vi "CAN Alerts.vi"(10 "RobotDriveDevRef":T1={"DevStatus"={"status"=FALSE, "code"=0, "source"=""}, "Motors[]"=[], "Square Inputs"=FALSE, "Max Output"=1.0}, 11 "CAN Talon List":string[](array[string])) -> ()   [LabVIEW 2014, in "hhVI.lvlib"]
doc: "Checks voltage of the PDV, roboRIO and all CAN Talon motor controllers. If the voltage on any of these it too low a dashboard message \"Voltage Alerts\" is sent."
uses:
  hhVI.lvlib
  <vilib>/Rock Robotics/Network Tables/SD Write String.vi
  <vilib>/Rock Robotics/WPI/PWM/WPI_PWMTransform_ConPane.ctl
  <vilib>/Rock Robotics/WPI/CAN/Jaguar/SubVIs/WPI_CANJaguar_ControlMode.ctl
  <vilib>/Rock Robotics/WPI/CAN/TalonSRX/WPI_CANTalonSRX_APIControlMode.ctl
  <vilib>/Rock Robotics/SystemInterfaces/Typedef/FPGA_TypedefDigitalModule.ctl
  <vilib>/Rock Robotics/SystemInterfaces/DIO/FPGA_DIOPWMChannel.ctl
  <vilib>/Rock Robotics/WPI/PWM/WPI_PWMDeadband.ctl
  <vilib>/Rock Robotics/WPI/MotorControl/WPI_MotorControlType.ctl
  <vilib>/Rock Robotics/WPI/MotorControl/WPI_MotorControlDeviceRef.ctl
  <vilib>/Rock Robotics/WPI/RobotDrive/WPI_RobotDriveDevRef.ctl
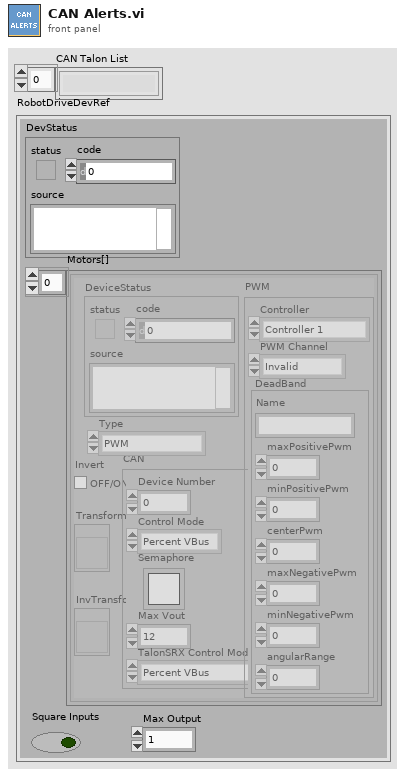
[diagram p1: front panel]
types:
  T1 = typedef "WPI_RobotDriveDevRef.ctl" = cluster{"DevStatus":errorcluster, "Motors[]":T2[], "Square Inputs":bool, "Max Output":dbl}
  T2 = typedef "WPI_MotorControlDeviceRef.ctl" = cluster{"DeviceStatus":errorcluster, "Type":T3, "PWM":cluster{"Controller":T4, "PWM Channel":T5, "DeadBand":T6}, "CAN":cluster{"Device Number":u8, "Control Mode":T7, "Semaphore":T8, "Max Vout":dbl, "TalonSRX Control Mode":T9}, "Invert":bool, "TransformRef":T10, "InvTransformRef":T10}
  T3 = typedef "WPI_MotorControlType.ctl" = enum16{"PWM", "CAN", "CANTalonSRX"}
  T4 = typedef "FPGA_TypedefDigitalModule.ctl" = enum16{"Controller 1"}
  T5 = typedef "FPGA_DIOPWMChannel.ctl" = enum8{"PWM 0", "PWM 1", "PWM 2", "PWM 3", "PWM 4", "PWM 5", "PWM 6", "PWM 7", "PWM 8", "PWM 9", "PWM MXP 0", "PWM MXP 1", "PWM MXP 2", "PWM MXP 3", "PWM MXP 4", "PWM MXP 5", "PWM MXP 6", "PWM MXP 7", "PWM MXP 8", "PWM MXP 9", "Invalid"}
  T6 = typedef "WPI_PWMDeadband.ctl" = cluster{"Name":string, "maxPositivePwm":i32, "minPositivePwm":i32, "centerPwm":i32, "maxNegativePwm":i32, "minNegativePwm":i32, "angularRange":u16}
  T7 = typedef "WPI_CANJaguar_ControlMode.ctl" = enum8{"Percent VBus", "Current", "Speed", "Position", "Voltage"}
  T8 = typedef "Semaphore RefNum" = refnum<k1>
  T9 = typedef "WPI_CANTalonSRX_APIControlMode.ctl" = enum8{"Percent VBus", "Speed", "Position", "Slave", "Unchanged / Invalid"}
  T10 = typedef "WPI_PWMTransform_ConPane.ctl" = refnum<vi>
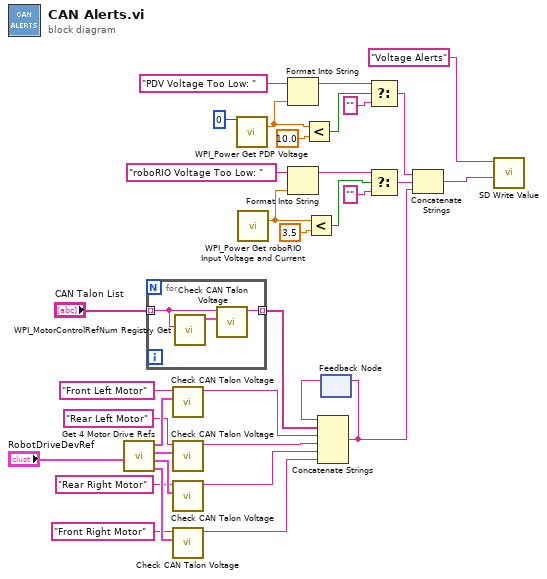
[diagram p0: block diagram]
diagram:
  n1 = call "Get 4 Motor Drive Refs.vi"("RobotDriveDevRef"="RobotDriveDevRef") -> ("FrontRightMotorControlDeviceRef"=w9:T2, "RearRightMotorControlDeviceRef"=w10:T2, "RearLeftMotorControlDeviceRef"=w11:T2, "FrontLeftMotorControlDeviceRef"=w13:T2)  [unwired: 7 in]
  n2 = for {
    tunnel: "CAN Talon List" -> [w36] mode=indexing
    tunnel: [w35] -> w19 mode=indexing
    n3 = call <vilib>:"WPI_MotorControlRefNum Registry Get.vi"("refnum name"=w36) -> ("MotorControlDevRef"=w37:T2)  [unwired: 9 in, 1 out]
    n4 = call "Check CAN Talon Voltage.vi"("CAN Talon SRX Ref"=w37, "Device Name"=w36) -> ("Error Message"=w35:string)  [unwired: 9 in]
  }
  n5 = call "Check CAN Talon Voltage.vi"("CAN Talon SRX Ref"=w13, "Device Name"="Front Left Motor") -> ("Error Message"=w12:string)  [unwired: 9 in]
  n6 = call "Check CAN Talon Voltage.vi"("CAN Talon SRX Ref"=w11, "Device Name"="Rear Left Motor") -> ("Error Message"=w7:string)  [unwired: 9 in]
  n7 = call "Check CAN Talon Voltage.vi"("CAN Talon SRX Ref"=w10, "Device Name"="Rear Right Motor") -> ("Error Message"=w3:string)  [unwired: 9 in]
  n8 = call "Check CAN Talon Voltage.vi"("CAN Talon SRX Ref"=w9, "Device Name"="Front Right Motor") -> ("Error Message"=w2:string)  [unwired: 9 in]
  n9 = call <vilib>:"WPI_Power Get PDP Voltage.vi"("Power Distribution Panel (0)"=u8 0) -> ("voltage (V)"=w27:dbl)  [unwired: 13 in, 1 out]
  n10 = call <vilib>:"WPI_Power Get roboRIO Input Voltage and Current.vi"() -> ("roboRIO input voltage (V)"=w14:dbl)  [unwired: 13 in, 2 out]
  n11 = Format Into String(initial string="PDV Voltage Too Low: ", w27) -> (resulting string=w25:string)  [unwired: 2 in, 1 out]
  n12 = Format Into String(initial string="roboRIO Voltage Too Low: ", w14) -> (resulting string=w20:string)  [unwired: 2 in, 1 out]
  n13 = Less?(x=w27, y=10.0) -> (x < y?=w32:bool)
  n14 = Less?(x=w14, y=3.5) -> (x < y?=w23:bool)
  n15 = feedback #1() -> (w18:string)  [unwired: 1 in]
  n16 = Concatenate Strings(w18, w19, w12, w7, w3, w2) -> (w16:string)
  n17 = feedback-in #1(w16) -> ()
  n18 = Select(t=w25, s=w32, f="") -> (s? t:f=w28:string)
  n19 = Select(t=w20, s=w23, f="") -> (s? t:f=w21:string)
  n20 = Concatenate Strings(w28, w21, w16) -> (w29:string)
  n21 = call-poly <vilib>:"SD Write Value.vi"("String"=w29, "Name"="Voltage Alerts") -> ()  [unwired: 8 in, 2 out]
